vi "listfiles2_TOP.vi"(8 "Error In":errorcluster) -> (0 "error out":errorcluster)   [LabVIEW 2014, in "LabVIEW Universal Transcriptor SD Card Library.lvlib"]
uses:
  LabVIEW Universal Transcriptor SD Card Library.lvlib
  <vilib>/LabVIEW Universal Transcriptor/LabVIEW to Arduino Transcriptor/Transcriptors/System API/Serial println string.vi
  <vilib>/LabVIEW Universal Transcriptor/LabVIEW to Arduino Transcriptor/Transcriptors/System API/System Serial Library Variables/System Serial Library Variables.lvlib
panel:
  out "String Buffer":string
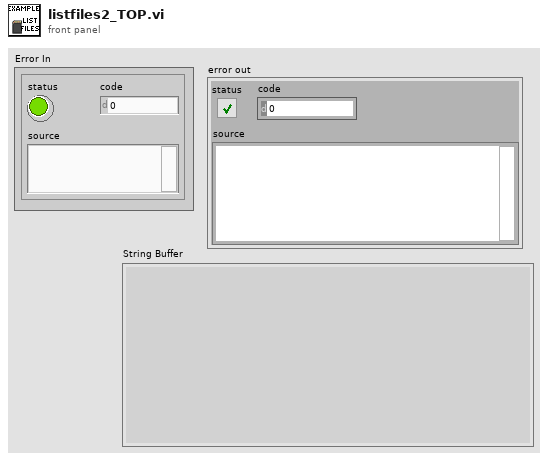
[diagram p1: front panel]
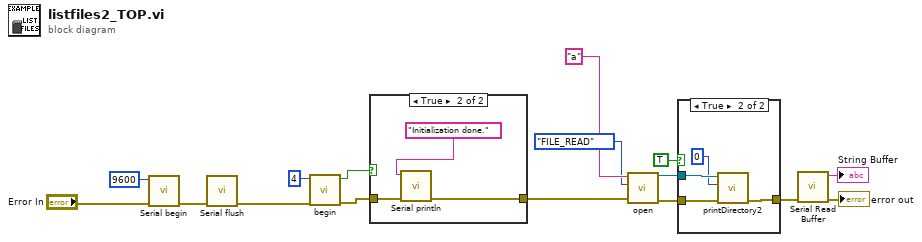
[diagram p0: block diagram]
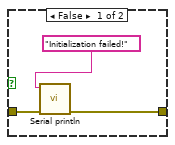
[diagram p3: hidden frame]
diagram:
  n1 = call <vilib>:"Serial begin.vi"("Error In"="Error In", "speed (Bd)"=9600) -> ("Error Out"=w2:errorcluster)  [unwired: 9 in]
  n2 = call <vilib>:"Serial flush.vi"("Error In"=w2) -> ("Error Out"=w1:errorcluster)  [unwired: 10 in]
  n3 = call "begin.vi"("Error In"=w1, "CS pin (optional)"=u8 4) -> ("Error Out"=w13:errorcluster, "success?"=w12:bool)  [unwired: 8 in]
  n4 = case shown="True" w12 {
    tunnel: w13 -> [w18 w21]
    tunnel: [w17 w20] -> w11
    frame False {
      n5 = call-poly <vilib>:"Serial println.vi"("Error In"=w18, "string in"="Initialization failed!" ("filepath")) -> ("Error Out"=w17:errorcluster)  [unwired: 9 in]
    }
    frame True {
      n6 = call-poly <vilib>:"Serial println.vi"("Error In"=w21, "string in"="Initialization done." ("filepath")) -> ("Error Out"=w20:errorcluster)  [unwired: 9 in]
    }
  }
  n7 = call "open.vi"("Error In"=w11, "mode"=enum16{"FILE_READ", "FILE_WRITE"}."FILE_READ", "filepath"="a") -> ("Error Out"=w8:errorcluster, "File out"=w7:refnum<class "File.lvclass">)  [unwired: 6 in, 1 out]
  n8 = case shown="True" TRUE {
    tunnel: w8 -> [w23 w27]
    tunnel: w7 -> [_ w26]
    tunnel: [w23 w24] -> w5
    frame False {
    }
    frame True {
      n9 = call "printDirectory2.vi"("Error In"=w27, "nested level"=u8 0, "file"=w26) -> ("Error Out"=w24:errorcluster)  [unwired: 8 in]
    }
  }
  n10 = call <vilib>:"Serial Read Buffer.vi"("Error In"=w5) -> ("Error Out"=→"error out":errorcluster, "String Buffer"=→"String Buffer":string)  [unwired: 9 in]
